vi "Pre Launch Init.vi"(11 "CS++SimMotor in":refnum<class "CS++SimMotor.lvclass">) -> (0 "error out":errorcluster, 3 "CS++SimMotor out":refnum<class "CS++SimMotor.lvclass">)   [LabVIEW 2015, in "CS++SimMotor.lvlib" / "CS++SimMotor.lvclass"]
doc: "(<B>Filename</B>: Actor Framework.lvlib:Actor.lvclass:Pre Launch Init.vi)\n\nDefines behavior that occurs after the Launch Actor method is invoked but before the actor's Actor Core method begins running.\n\nThe Pre Launch Init method is guaranteed to finish before the Launch Actor method returns to its caller and before the actor itself receives any messages. Any references that the Pre Launch Init method obtains are guaranteed to have the same lifetime as the actor itself. Any errors that the Pre Launch Init method returns will abort the launch.\n\nBy default, this method does nothing. A descendant class may override it to define behavior."
uses:
  CS++SimMotor.lvclass
  CS++SimMotor.lvclass/CS++SimMotor.ctl
  CSPP_DeviceBase/CS++Motor/CS++Motor.lvclass
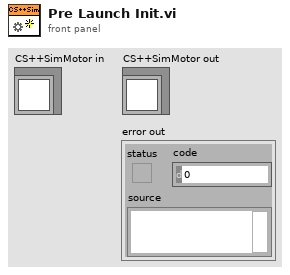
[diagram p1: front panel]
types:
  T1 = cluster{"AxisNumber":u8, "Raw-Position":dbl, "Enum":enum16{"RelativeMovement", "AbsoluteMovement", "Stop", "ReferenceMovement"}}
  T2 = cluster{"Stop":refnum<user-event>, "Pos Update":refnum<user-event>, "Reset":refnum<user-event>}
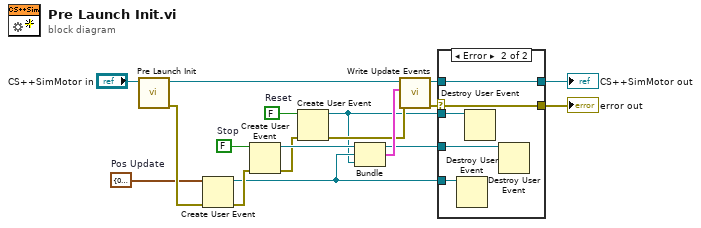
[diagram p0: block diagram]
diagram:
  w4 = FALSE  # Reset
  w5 = T1 {"AxisNumber"=0, "Raw-Position"=0.0, "Enum"=enum."RelativeMovement"}  # Pos Update
  w11 = FALSE  # Stop
  n1 = call-parent "Pre Launch Init.vi"("CS++Motor in"="CS++SimMotor in") -> ("error out"=w6:errorcluster, "CS++Motor out"=w16:refnum<class "CS++SimMotor.lvclass">)  [unwired: 9 in]
  n2 = Create User Event(user event datatype=w5, error in=w6) -> (user event=w7:refnum<user-event>, error out=w8:errorcluster)
  n3 = Create User Event(user event datatype=w11, error in=w8) -> (user event=w9:refnum<user-event>, error out=w3:errorcluster)
  n4 = Create User Event(user event datatype=w4, error in=w3) -> (user event=w1:refnum<user-event>, error out=w2:errorcluster)
  n5 = Bundle("Stop"=w9, "Pos Update"=w7, "Reset"=w1) -> (w10:T2)  [unwired: 1 in]
  n6 = call "Write Update Events.vi"("error in (no error)"=w2, "Update Events"=w10, "CS++SimMotor in"=w16) -> ("error out"=w15:errorcluster, "CS++SimMotor out"=w12:refnum<class "CS++SimMotor.lvclass">)  [unwired: 7 in]
  n7 = case shown="Error" w15 {
    selector: w15 -> [w19 w23]
    tunnel: [w19 w23] -> w14
    tunnel: [w18 w24] -> w13
    tunnel: w12 -> [w18 w24]
    tunnel: w9 -> [_ w22]
    tunnel: w7 -> [_ w21]
    tunnel: w1 -> [_ w20]
    frame No Error {
    }
    frame Error {
      n8 = Destroy User Event(user event=w21) -> ()  [unwired: 1 in, 1 out]
      n9 = Destroy User Event(user event=w20) -> ()  [unwired: 1 in, 1 out]
      n10 = Destroy User Event(user event=w22) -> ()  [unwired: 1 in, 1 out]
    }
  }
  "error out" <- w14
  "CS++SimMotor out" <- w13
